vi "API get Sensor Statue.vi"(10 "array input":i32[](array[numeric])) -> (2 "array output":i32[](array[numeric]), 3 "return value":bool)   [LabVIEW 2011, in "API DYM.lvlib"]
uses:
  API DYM.lvlib
  DyMechnicalPlatform.dll
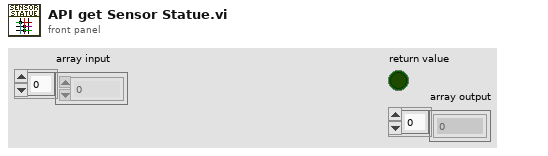
[diagram p1: front panel]
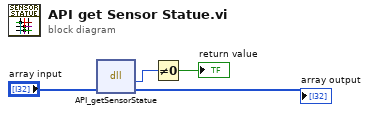
[diagram p0: block diagram]
diagram:
  n1 = dll-call lib="PTH1Xabs D可重构机电平台项目DemoLabViewDYSYSAPIDyMechnicalPlatform.dll" fn="API_getSensorStatue"("SensorStatueArray"="array input") -> ("返回类型"=w3:i32, "SensorStatueArray"=→"array output":i32[])  [unwired: 3 in, 2 out]
  n2 = Not Equal To 0?(x=w3) -> (x != 0?=→"return value":bool)
